vi "Change Decoration Color.vi"(0 "This VI":refnum<vi>, 3 "Colors:BG Color":u32) -> (10 "error out":errorcluster)   [LabVIEW 2020]
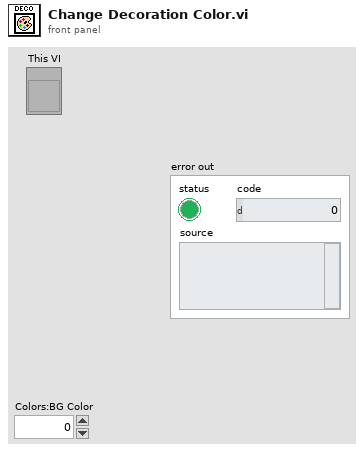
[diagram p1: front panel]
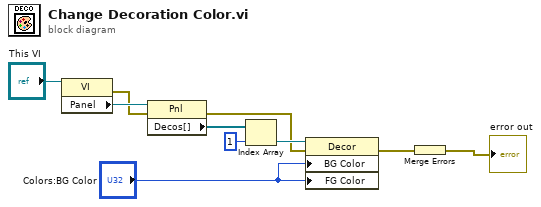
[diagram p0: block diagram]
diagram:
  n1 = property class="VI"(reference="This VI") -> (error out=w9:errorcluster, "Panel"=w10:refnum<vi>)  [unwired: 1 in, 1 out]
  n2 = property class="Pnl"(reference=w10, error in=w9) -> (error out=w5:errorcluster, "Decos[]"=w8:refnum<vi>[])  [unwired: 1 out]
  n3 = Index Array(array=w8, index=1) -> (element=w6:refnum<vi>)
  n4 = property class="Decor"(reference=w6, error in=w5, "BG Color"="Colors:BG Color", "FG Color"="Colors:BG Color") -> (error out=w3:errorcluster)  [unwired: 1 out]
  n5 = Merge Errors(w3) -> (→"error out":errorcluster)
